vi "Bind RPC adas_NodeCustomService_SetExample_1.vi"(11 "gRPCid server in":T3) -> (0 "error out":errorcluster, 1 "adas_NodeCustomService_SetExample_1 Internal UE":T2, 2 "adas_NodeCustomService_SetExample_1 gRPC UE":T1, 3 "gRPCid server out":T3)   [LabVIEW 2019, in "Example_1_server.lvlib" / "NodeCustomService.lvclass"]
uses:
  NodeCustomService.lvclass
  616620f9-6bbe-466a-af51-04bcc3596ea0.vi
  <vilib>/gRPC/LabVIEW gRPC Library/Shared/grpcId.ctl
  <vilib>/gRPC/LabVIEW gRPC Library/grpc-lvsupport-release.lvlib
  <vilib>/gRPC/LabVIEW gRPC Library/Server API/typeDefs/gRPCId Cluster.ctl
  typeDefs/Server Internal Message.ctl
  typeDefs/Server Internal Message UE.ctl
  <vilib>/gRPC/LabVIEW gRPC Library/Server API/typeDefs/gRPCId Cluster UE.ctl
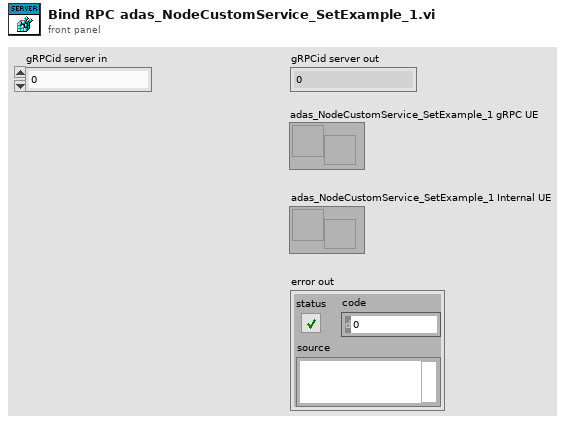
[diagram p1: front panel]
types:
  T1 = typedef "grpc-lvsupport-release.lvlib/gRPCId Cluster UE.ctl" = refnum<user-event>
  T2 = typedef "Example_1_server.lvlib/NodeCustomService.lvclass/Server Internal Message UE.ctl" = refnum<user-event>
  T3 = typedef "grpc-lvsupport-release.lvlib/grpcId.ctl" = u64
  T4 = typedef "Example_1_server.lvlib/NodeCustomService.lvclass/Server Internal Message.ctl" = cluster{"Command":string, "Data":variant}
  T5 = typedef "grpc-lvsupport-release.lvlib/gRPCId Cluster.ctl" = cluster{"gRPCid":T3}
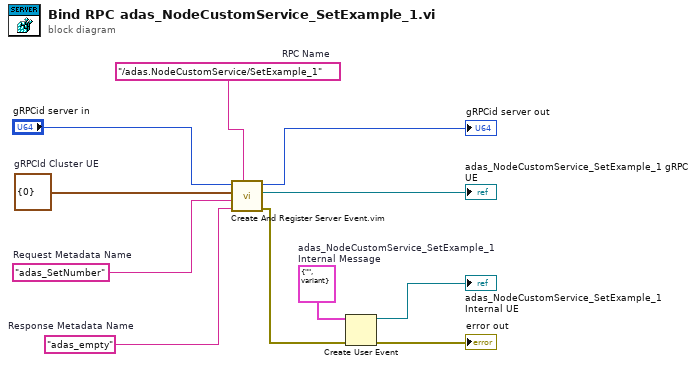
[diagram p0: block diagram]
diagram:
  w5 = T4 {"Command"="", "Data"=variant}  # adas_NodeCustomService_SetExample_1 Internal Message
  w8 = "adas_empty"  # Response Metadata Name
  w11 = T5 {"gRPCid"=0}  # gRPCId Cluster UE
  w9 = "adas_SetNumber"  # Request Metadata Name
  w10 = "/adas.NodeCustomService/SetExample_1"  # RPC Name
  n1 = call "Create And Register Server Event.vim"("Method name"=w10, "Response Metadata Name"=w8, "Request Metadata Name"=w9, "event in"=w11, "gRPCid server in"="gRPCid server in") -> ("error out"=w4:errorcluster, "event"=→"adas_NodeCustomService_SetExample_1 gRPC UE":refnum<user-event>, "gRPCid server out"=→"gRPCid server out":T3)  [unwired: 4 in]
  n2 = Create User Event(user event datatype=w5, error in=w4) -> (user event=→"adas_NodeCustomService_SetExample_1 Internal UE":refnum<user-event>, error out=→"error out":errorcluster)
